vi "Generate_pseudo_unique_filename.vi"(10 "Optional iterator":i32, 11 "file type(.jpg)":T1) -> (1 "root filename":string, 2 "temp directory":path, 3 "generated path":path)   [LabVIEW 2017, in "NI_ReportGenerationCore.lvlib"]
uses:
  <vilib>/Utility/NIReport.llb/NI_ReportGenerationCore.lvlib
  <vilib>/printing/ReportDocExtensions.llb/File_types_for_reports.ctl
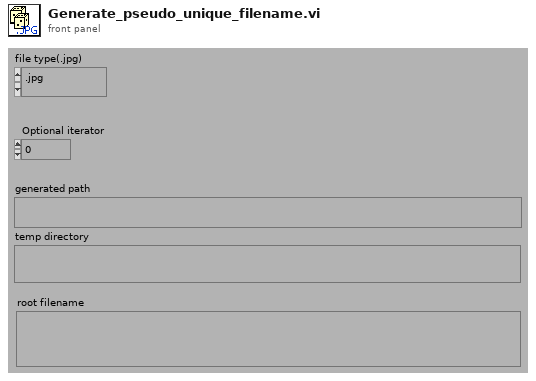
[diagram p1: front panel]
types:
  T1 = typedef "NI_ReportGenerationCore.lvlib/File_types_for_reports.ctl" = enum16{".jpg", ".png", ".html", ".gif"}
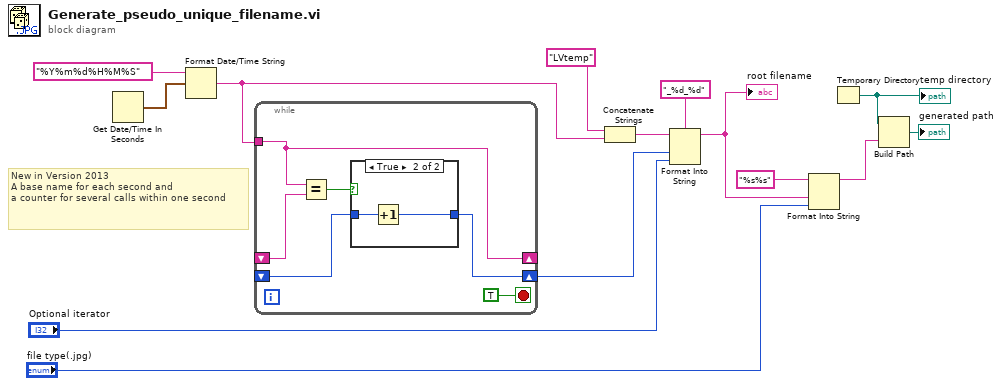
[diagram p0: block diagram]
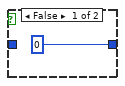
[diagram p2: hidden frame]
diagram:
  # "New in Version 2013\nA base name for each second and \na counter for several calls within one second"
  n1 = Get Date/Time In Seconds() -> (seconds since 1Jan1904=w6:timestamp)
  n2 = Format Date/Time String(time format string (%c)="%Y%m%d%H%M%S", seconds (now)=w6) -> (date/time string=w2:string)  [unwired: 1 in]
  n3 = while {
    tunnel: w2 -> [w17]
    shift-right: [w17] -> _
    shift-left: _ -> [w19]
    shift-right: [w16] -> w1
    shift-left: _ -> [w15]
    stop <- TRUE stop-if-true
    n4 = Equal?(x=w17, y=w19) -> (x = y?=w18:bool)
    n5 = case shown="True" w18 {
      tunnel: [0 ("Counter") w22] -> w16
      tunnel: w15 -> [_ w23]
      frame False {
      }
      frame True {
        n6 = Increment(x=w23) -> (x+1=w22:i32)
      }
    }
  }
  n7 = Concatenate Strings("LVtemp" ("string"), w2) -> (w4:string)
  n8 = Format Into String(format string="_%d_%d" ("Format String"), initial string=w4, w1, "Optional iterator") -> (resulting string=w8:string)  [unwired: 1 in, 1 out]
  "root filename" <- w8
  n9 = Format Into String(format string="%s%s", w8, "file type(.jpg)") -> (resulting string=w9:string)  [unwired: 2 in, 1 out]
  n10 = Temporary Directory() -> (w14:path)
  "temp directory" <- w14
  n11 = Build Path(base path=w14, name or relative path=w9) -> (appended path=→"generated path":path)
